vi "Read channels.vi"(8 "error in":errorcluster, 11 "TEC configuration in":refnum<class "TEC configuration.lvclass">) -> (0 "error out":errorcluster, 2 "channels":refnum<class "TBM channel.lvclass">[](array[class]), 3 "TEC configuration out":refnum<class "TEC configuration.lvclass">)   [LabVIEW 2013, in "TEC configuration.lvclass"]
uses:
  TEC configuration.lvclass
  <vilib>/NI/Tag Bus Module Framework/channel/TBM channel.lvclass
  TEC configuration.lvclass/TEC configuration.ctl
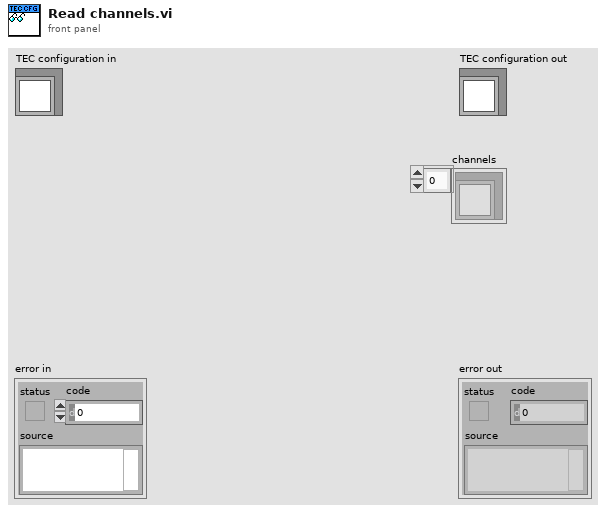
[diagram p1: front panel]
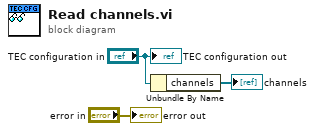
[diagram p0: block diagram]
diagram:
  n1 = Unbundle By Name("TEC configuration in") -> ("channels"=→"channels":refnum<class "TBM channel.lvclass">[])
  "error out" <- "error in"
  "TEC configuration out" <- "TEC configuration in"
